vi "BigIntIsLess.vi"(1 "b":cluster{"Boolean":bool, "Array":u64[]}, 2 "a":cluster{"Boolean":bool, "Array":u64[]}) -> (0 "a < b":bool)   [LabVIEW 2023]
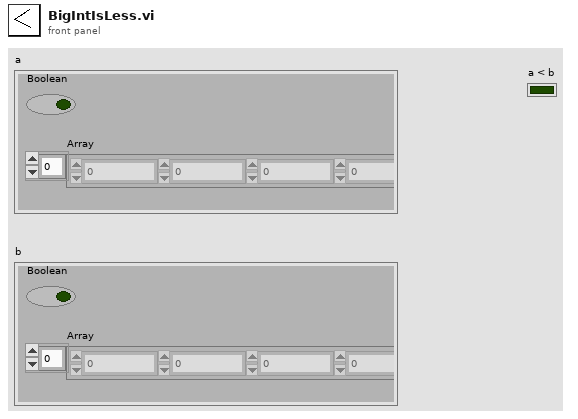
[diagram p1: front panel]
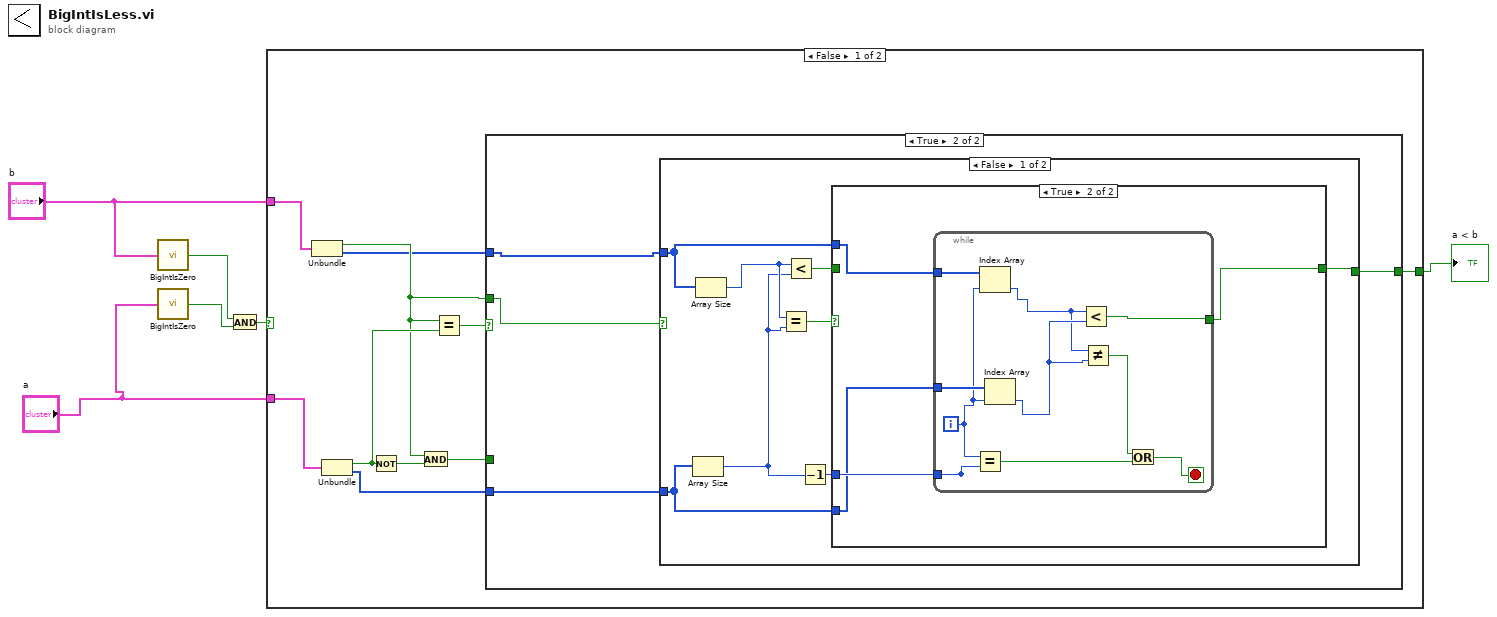
[diagram p0: block diagram]
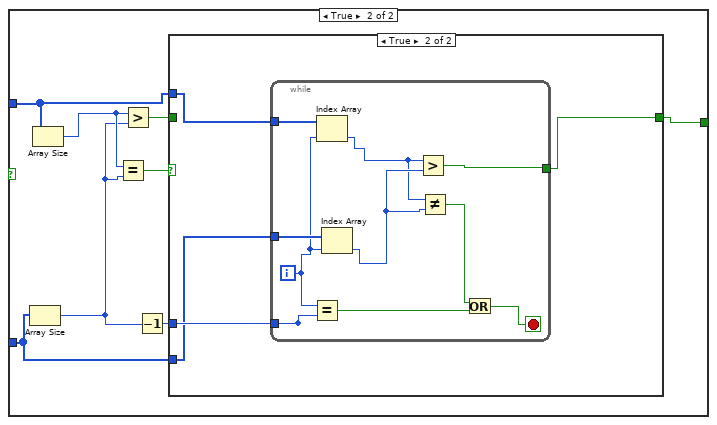
[diagram p4: hidden frame]
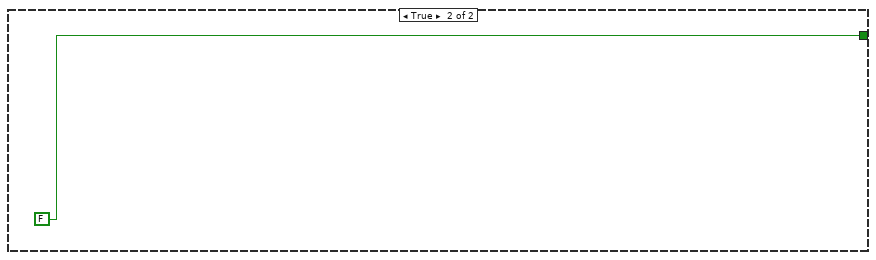
[diagram p6: hidden frame]
diagram:
  n1 = call "BigIntIsZero.vi"("a"="b") -> ("a = 0"=w6:bool)
  n2 = call "BigIntIsZero.vi"("a"="a") -> ("a = 0"=w5:bool)
  n3 = And(x=w6, y=w5) -> (x .and. y?=w4:bool)
  n4 = case shown="False" w4 {
    tunnel: [w11 FALSE] -> w1
    tunnel: "b" -> [w10 _]
    tunnel: "a" -> [w9 _]
    frame False {
      n5 = Unbundle(w10) -> ("Boolean"=w13:bool, "Array"=w8:u64[])
      n6 = Unbundle(w9) -> ("Boolean"=w15:bool, "Array"=w7:u64[])
      n7 = Not(x=w15) -> (.not. x?=w16:bool)
      n8 = And(x=w13, y=w16) -> (x .and. y?=w12:bool)
      n9 = Equal?(x=w13, y=w15) -> (x = y?=w14:bool)
      n10 = case shown="True" w14 {
        tunnel: w13 -> [_ w21]
        tunnel: [w17 w20] -> w11
        tunnel: w12 -> [w17 _]
        tunnel: w8 -> [_ w19]
        tunnel: w7 -> [_ w18]
        frame False {
        }
        frame True {
          n11 = case shown="False" w21 {
            tunnel: [w22 w49] -> w20
            tunnel: w19 -> [w24 w45]
            tunnel: w18 -> [w23 w46]
            frame False {
              n12 = Array Size(array=w23) -> (size(s)=w25:i32)
              n13 = Array Size(array=w24) -> (size(s)=w26:i32)
              n14 = Equal?(x=w26, y=w25) -> (x = y?=w29:bool)
              n15 = Less?(x=w26, y=w25) -> (x < y?=w28:bool)
              n16 = Decrement(x=w25) -> (x-1=w27:i32)
              n17 = case shown="True" w29 {
                tunnel: w28 -> [w30 _]
                tunnel: [w30 w33] -> w22
                tunnel: w27 -> [_ w34]
                tunnel: w23 -> [_ w32]
                tunnel: w24 -> [_ w31]
                frame False {
                }
                frame True {
                  n18 = while {
                    tunnel: [w44] -> _
                    tunnel: w34 -> [w44]
                    tunnel: [w41] -> w33
                    tunnel: w32 -> [w38]
                    tunnel: w31 -> [w39]
                    i -> [w37]
                    stop <- w42 stop-if-true
                    n19 = Equal?(x=w37, y=w44) -> (x = y?=w43:bool)
                    n20 = Index Array(array=w39, index=w37) -> (element=w35:u64)
                    n21 = Index Array(array=w38, index=w37) -> (element=w36:u64)
                    n22 = Less?(x=w35, y=w36) -> (x < y?=w41:bool)
                    n23 = Not Equal?(x=w35, y=w36) -> (x != y?=w40:bool)
                    n24 = Or(x=w40, y=w43) -> (x .or. y?=w42:bool)
                  }
                }
              }
            }
            frame True {
              n25 = Array Size(array=w46) -> (size(s)=w47:i32)
              n26 = Array Size(array=w45) -> (size(s)=w48:i32)
              n27 = Equal?(x=w48, y=w47) -> (x = y?=w52:bool)
              n28 = Greater?(x=w48, y=w47) -> (0:w51:bool)
              n29 = Decrement(x=w47) -> (x-1=w50:i32)
              n30 = case shown="True" w52 {
                tunnel: w51 -> [w53 _]
                tunnel: [w53 w56] -> w49
                tunnel: w50 -> [_ w57]
                tunnel: w46 -> [_ w55]
                tunnel: w45 -> [_ w54]
                frame False {
                }
                frame True {
                  n31 = while {
                    tunnel: [w67] -> _
                    tunnel: w57 -> [w67]
                    tunnel: [w64] -> w56
                    tunnel: w55 -> [w61]
                    tunnel: w54 -> [w62]
                    i -> [w60]
                    stop <- w65 stop-if-true
                    n32 = Equal?(x=w60, y=w67) -> (x = y?=w66:bool)
                    n33 = Index Array(array=w62, index=w60) -> (element=w58:u64)
                    n34 = Index Array(array=w61, index=w60) -> (element=w59:u64)
                    n35 = Greater?(x=w58, y=w59) -> (0:w64:bool)
                    n36 = Not Equal?(x=w58, y=w59) -> (x != y?=w63:bool)
                    n37 = Or(x=w63, y=w66) -> (x .or. y?=w65:bool)
                  }
                }
              }
            }
          }
        }
      }
    }
    frame True {
    }
  }
  "a < b" <- w1
